vi "Configure Flow Rate.vi"(5 "Retry Attempts (0)":i32 min=0, 7 "Fast Comms (F)":bool, 8 "error in":errorcluster, 10 "Flow Input (ml/min)":dbl, 11 "VISA resource name":refnum<visa-resource-name>) -> (0 "error out":errorcluster, 2 "Flow Output":dbl, 3 "VISA resource name out":refnum<visa-resource-name>)   [LabVIEW 2020, in "ChromTech MX-Class Drivers.lvlib"]
doc: "Configures the flow rate using up to 5 digits. If the entered value exceeds the maximum allowable flow rate of the pump, the flow rate will be automatically set to the maximum allowable flow rate. The maximum allowable flow rate can be found using the Get Maximum Flow Rate VI and the current flow rate can be found using the Get Current Flow Rate VI or Get Current Conditions VI"
uses:
  <instrlib>/RxnRover/ChromtechNextGenDriver/ChromTech MX-Class Drivers.lvlib
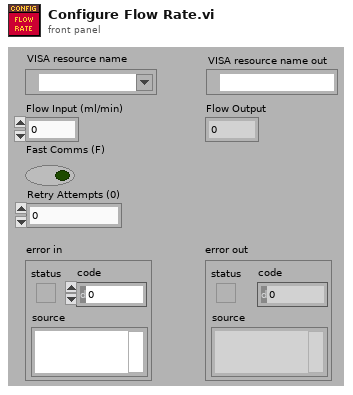
[diagram p1: front panel]
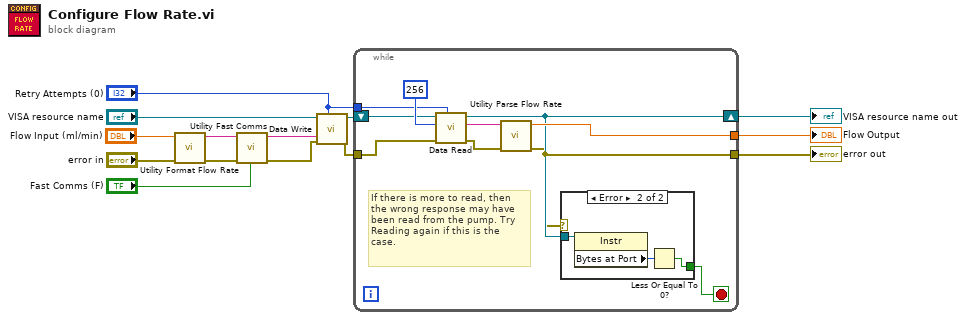
[diagram p0: block diagram]
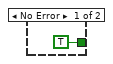
[diagram p2: hidden frame]
diagram:
  n1 = call <instrlib>:"Utility Format Flow Rate.vi"("error in (no error)"="error in", "Flow Rate"="Flow Input (ml/min)") -> ("error out"=w9:errorcluster, "Formatted Flow Rate"=w8:string)  [unwired: 8 in]
  n2 = call <instrlib>:"Utility Fast Comms.vi"("Fast Comms"="Fast Comms (F)", "Command"=w8) -> ("Fast Command"=w6:string)  [unwired: 9 in]
  n3 = call <instrlib>:"Data Write.vi"("Retry Attempts (0)"="Retry Attempts (0)", "error in (no error)"=w9, "Command"=w6, "VISA Refnum in"="VISA resource name") -> ("error out"=w12:errorcluster, "VISA Refnum out"=w4:refnum<visa-resource-name>)  [unwired: 6 in]
  n4 = while {
    tunnel: [w20] -> w7
    tunnel: "Retry Attempts (0)" -> [w17]
    shift-right: [w16] -> w2
    shift-left: w4 -> [w18]
    tunnel: w12 -> [w23]
    tunnel: [w15] -> w1
    stop <- w14 stop-if-true
    # "If there is more to read, then\nthe wrong response may have\nbeen read from the pump. Try\nReading again if this is the\ncase."
    n5 = call <instrlib>:"Data Read.vi"("Retry Attempts (0)"=w17, "error in (no error)"=w23, "Bytes to read"=256, "VISA Refnum in"=w18) -> ("error out"=w19:errorcluster, "read buffer"=w21:string, "VISA Refnum out"=w16:refnum<visa-resource-name>)  [unwired: 5 in]
    n6 = call <instrlib>:"Utility Parse Flow Rate.vi"("error in (no error)"=w19, "String"=w21) -> ("error out"=w15:errorcluster, "Numeric"=w20:dbl)  [unwired: 8 in]
    n7 = case shown="Error" w15 {
      tunnel: w16 -> [_ w27]
      tunnel: [TRUE w25] -> w14
      frame No Error {
      }
      frame Error {
        n8 = property class="Instr"(reference=w27) -> ("Bytes at Port"=w26:u32)  [unwired: 1 in, 2 out]
        n9 = Less Or Equal To 0?(x=w26) -> (x <= 0?=w25:bool)
      }
    }
  }
  "VISA resource name out" <- w2
  "error out" <- w1
  "Flow Output" <- w7
